vi "Initialize.vi"() -> (1 "Grid out":refnum<class "Grid.lvclass">, 2 "Synapses out":refnum<class "Synapses.lvclass">, 3 "Cerebellum out":refnum<class "Cerebellum.lvclass">, 4 "error out":errorcluster)   [LabVIEW 2016, in "Cerebellum.lvclass"]
doc: "Load/Create the flattened XML files for the Grid/Synapses/AER and plot it"
uses:
  Cerebellum.lvclass
  Cube/Grid.lvclass
  Controls/SM load Cere.ctl
  <vilib>/Utility/xml.llb/Read From XML File(string).vi
  Controls/Type of Neuron.ctl
  Synapses/Synapses.lvclass
  AER/AER.lvclass
  Neuron/Neuron.lvclass
panel:
  out "AER file path":path
  in  "Right":bool
  in  "Left":bool
  out "Syn ok?":bool
  in  "New AER":bool
  in  "Load AER":bool
  out "AER Loaded":string
  in  "3 - AER":i32(listbox)
  in  "Plot AER":bool
  in  "Plot Grid":bool
  in  "accept":bool
  out "Synapses Loaded":string
  out "Grid ok?":bool
  in  "New Synapses":bool
  in  "Load Synapses":bool
  in  "2 - Synapses":i32(listbox)
  out "Grid Loaded":string
  out "progress 2":dbl
  out "Preview":string
  in  "New Grid":bool
  in  "Cancel":bool
  in  "Load Grid":bool
  in  "1 - Grid":i32(listbox)
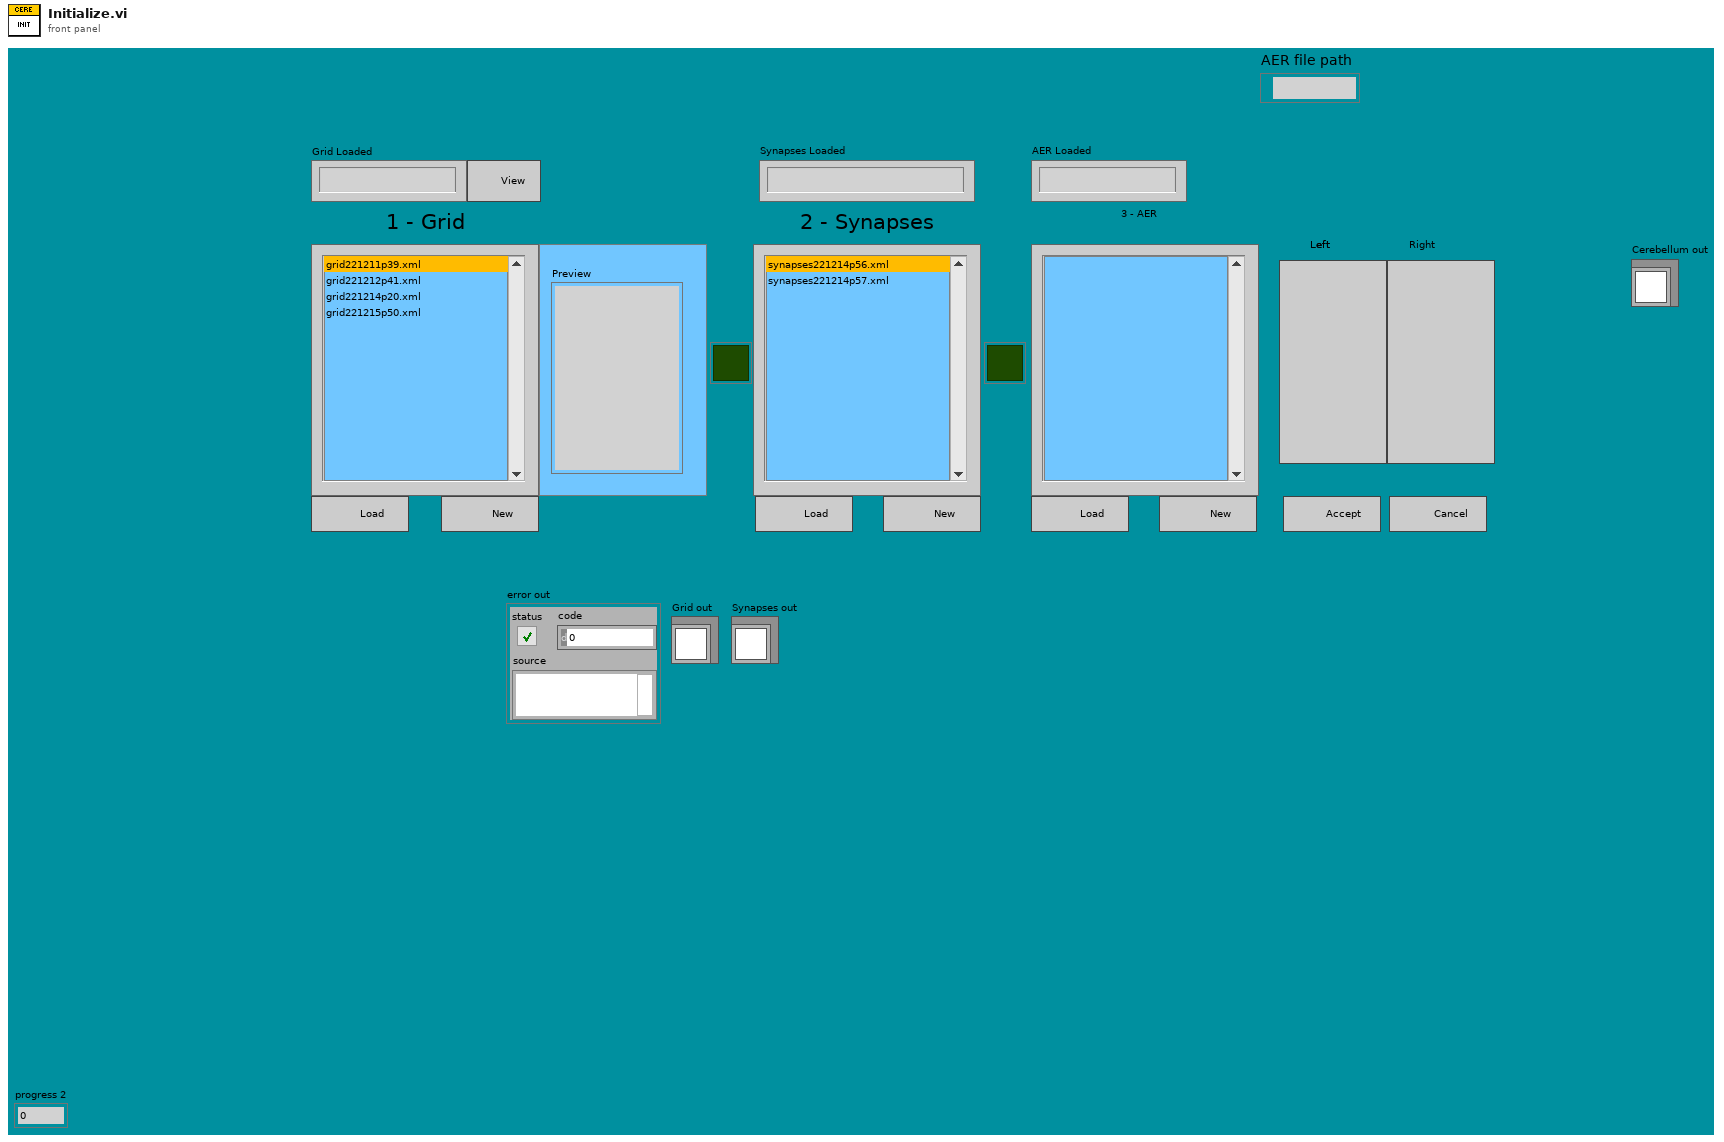
[diagram p1: front panel]
types:
  T1 = enum16{"open", "replace", "create", "open or create", "replace or create", "replace or create with confirmation"}
  T2 = typedef "SM load Cere.ctl" = enum16{"Create Grid", "Load Grid", "Create Synapses", "Load Synapses", "Cancel", "Update Lists", "accept", "Plot Grid", "Plot AER", "Load AER", "Create AER", "ToRightHem", "ToLeftHem"}
  T3 = typedef "Type of Neuron.ctl" = enum16{"MF", "BA", "GO", "GC", "PC", "LU", "Glia (Dummy)"}
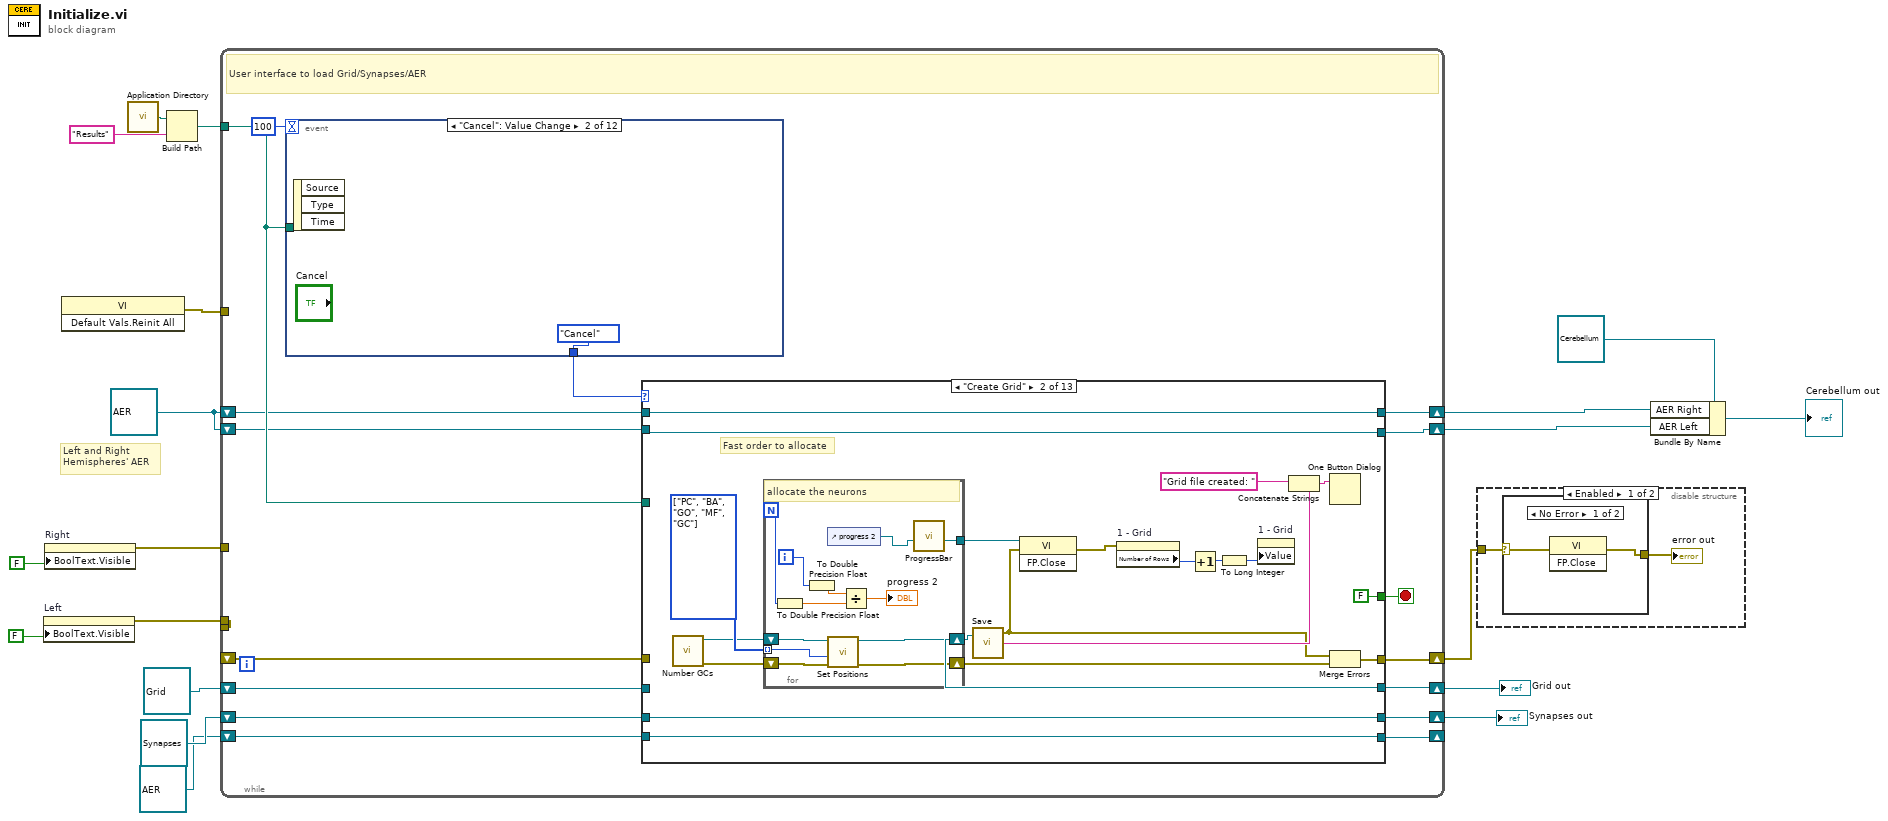
[diagram p0: block diagram]
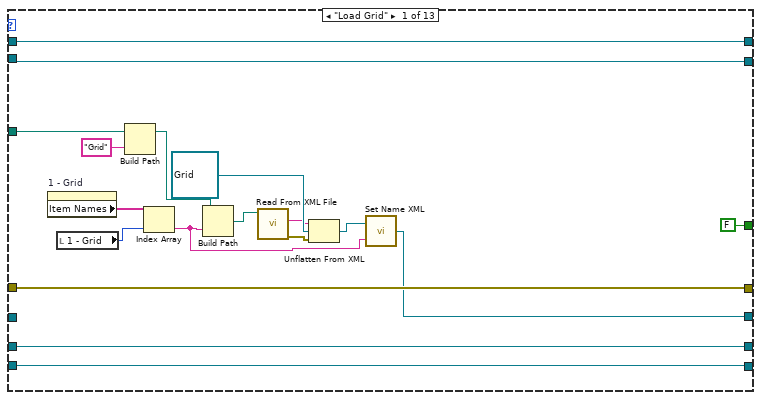
[diagram p4: hidden frame]
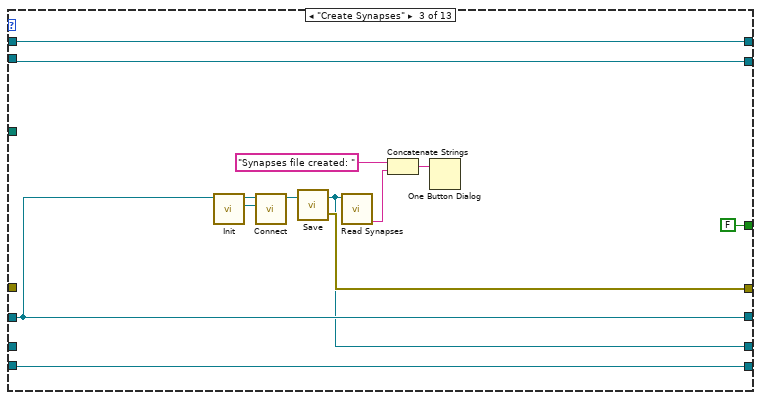
[diagram p5: hidden frame]
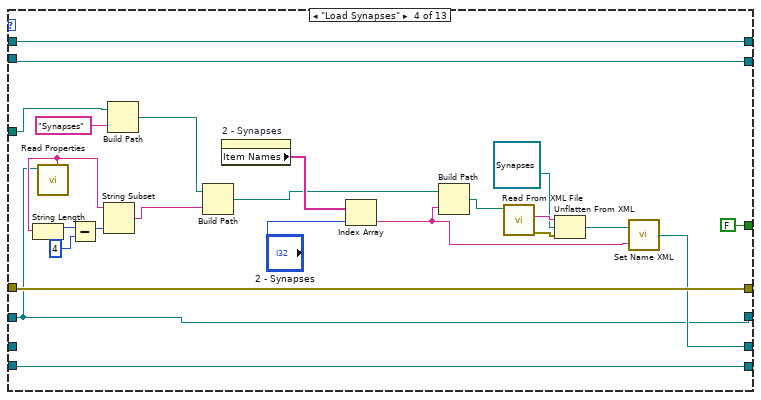
[diagram p6: hidden frame]
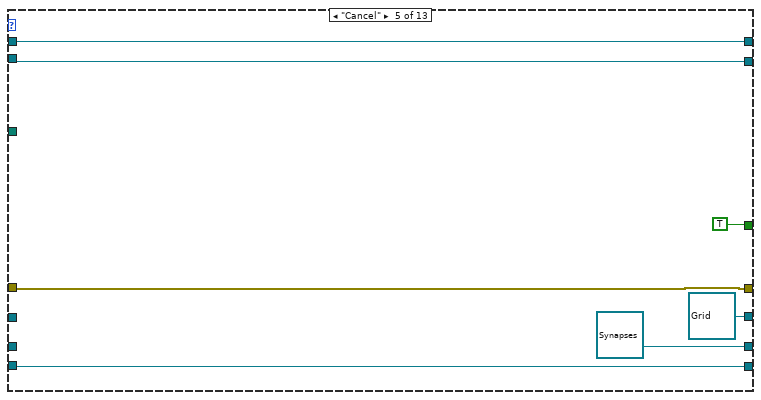
[diagram p7: hidden frame]
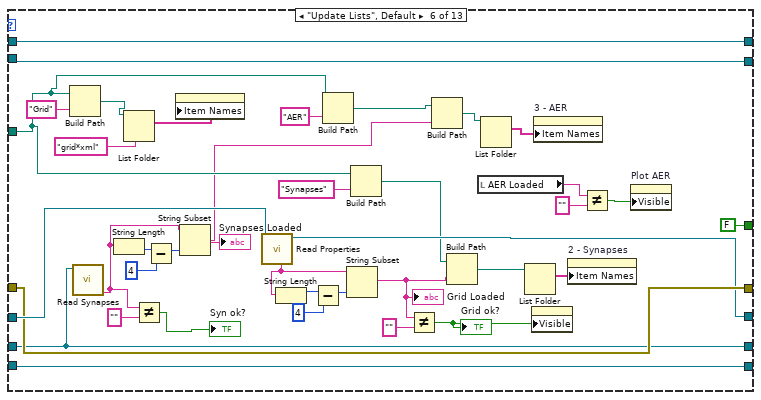
[diagram p8: hidden frame]
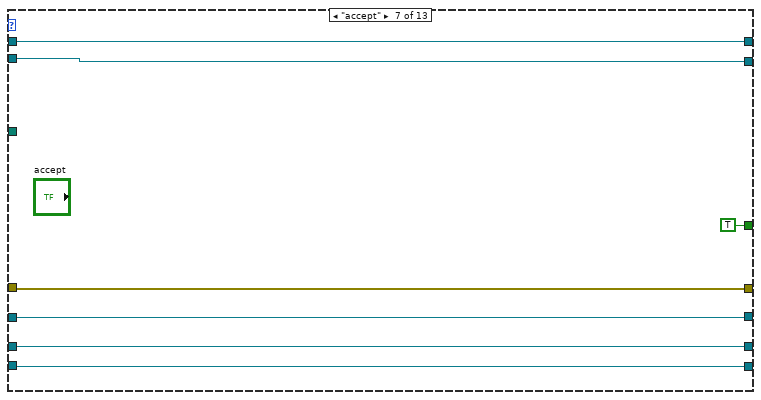
[diagram p9: hidden frame]
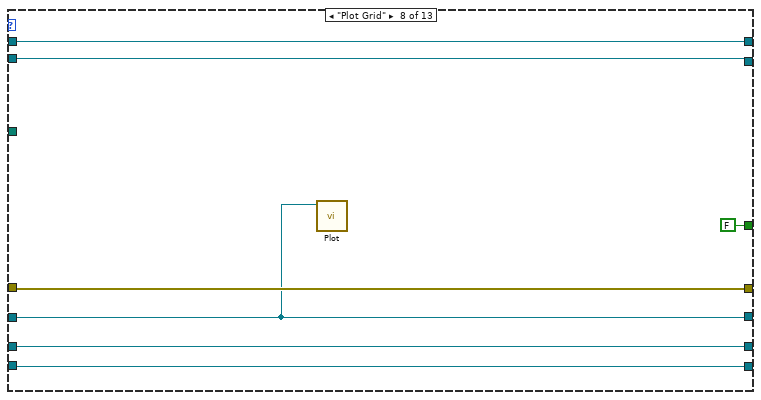
[diagram p10: hidden frame]
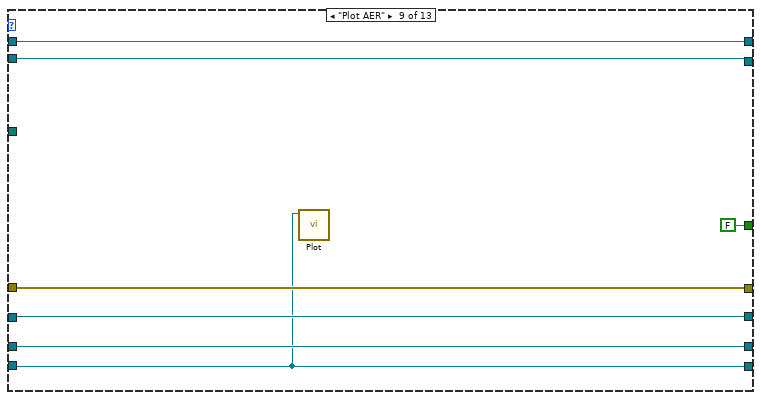
[diagram p11: hidden frame]
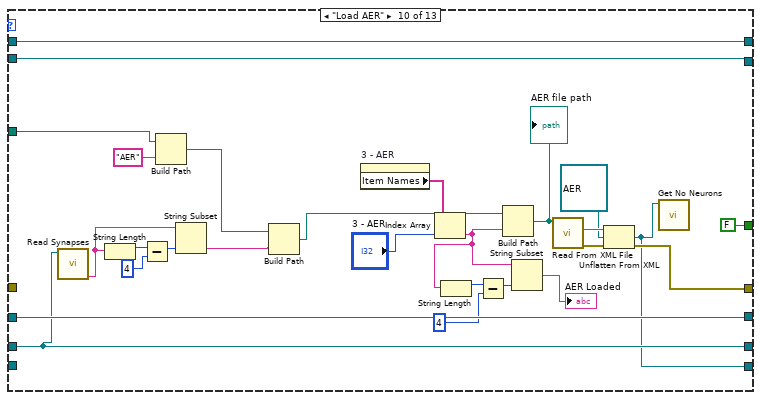
[diagram p12: hidden frame]
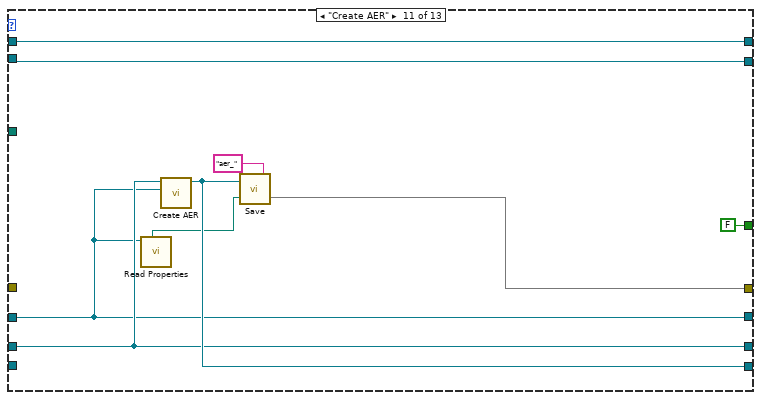
[diagram p13: hidden frame]
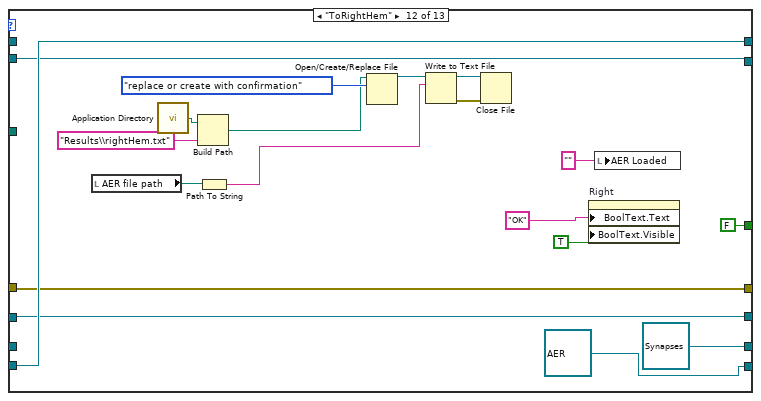
[diagram p14: hidden frame]
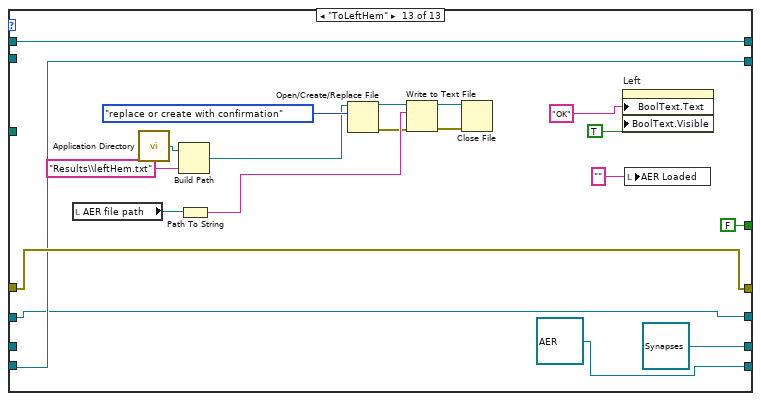
[diagram p15: hidden frame]
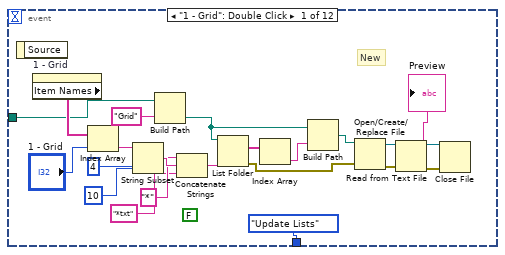
[diagram p16: hidden frame]
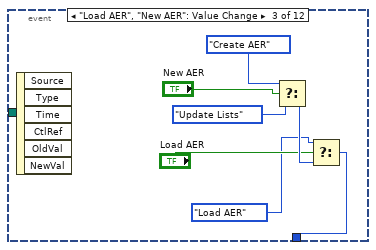
[diagram p17: hidden frame]
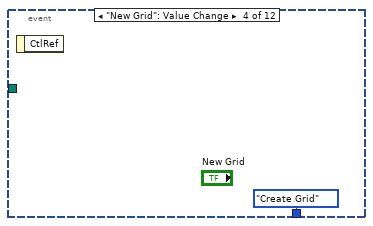
[diagram p18: hidden frame]
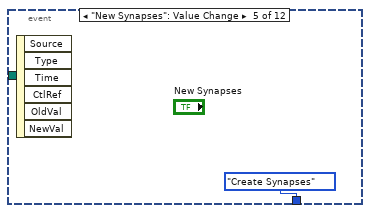
[diagram p19: hidden frame]
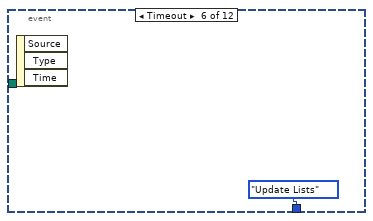
[diagram p20: hidden frame]
diagram:
  w9 = refnum<class "AER.lvclass"> refnum ("AER.lvclass")
  # "Left and Right\nHemispheres' AER"
  n1 = property on="Left" class="Bool (strict)"("BoolText.Visible"=FALSE ("Boolean Text.Visible")) -> (error out=w6:errorcluster)  [unwired: 2 in, 1 out]
  n2 = property on="Right" class="Bool (strict)"("BoolText.Visible"=FALSE ("Boolean Text.Visible")) -> (error out=w5:errorcluster)  [unwired: 2 in, 1 out]
  n3 = invoke class="VI" method="Default Vals.Reinit All"() -> (error out=w19:errorcluster)  [unwired: 3 in, 2 out]
  n4 = call <vilib>:"Application Directory.vi"() -> ("Application Directory"=w15:path)
  n5 = Build Path(base path=w15, name or relative path="Results") -> (appended path=w13:path)
  n6 = while {
    tunnel: w19 -> [_]
    shift-right: [w36] -> w18
    shift-left: refnum<class "Grid.lvclass"> refnum ("Cube out") -> [w33]
    shift-right: [w35] -> w16
    shift-left: _ -> [w34]
    tunnel: w13 -> [w32]
    shift-right: [w28] -> w11
    shift-left: refnum<class "Synapses.lvclass"> refnum ("Synapses out") -> [w27]
    shift-right: [w26] -> _
    shift-left: refnum<class "AER.lvclass"> refnum ("AER.lvclass") -> [w25]
    shift-right: [w22] -> w1
    shift-left: w9 -> [w21]
    shift-right: [w23] -> w2
    shift-left: w9 -> [w24]
    tunnel: [w20] -> _
    tunnel: w6 -> [w20]
    tunnel: w5 -> [_]
    stop <- w30 stop-if-true
    # "User interface to load Grid/Synapses/AER"
    n7 = event shown="[1] \"Cancel\": Value Change" {
      selector: _ -> [_ _ _ _ _ _ _ _ _ _ _ _]
      dyn-events: _ -> [_ _ _ _ _ _ _ _ _ _ _ _]
      timeout: 100 -> [_ _ _ _ _ _ _ _ _ _ _ _]
      tunnel: w32 -> [w268 _ _ _ _ _ _ _ _ _ _ _]
      tunnel: [SM_load_Cere."Update Lists" SM_load_Cere."Cancel" w288 SM_load_Cere."Create Grid" SM_load_Cere."Create Synapses" SM_load_Cere."Update Lists" SM_load_Cere."Load Synapses" SM_load_Cere."accept" w301 w307 SM_load_Cere."Load Grid" SM_load_Cere."Cancel"] -> w31
      event "1 - Grid": Double Click {
        (unwired) FALSE ("New")
        # "New"
        n8 = event-data() -> ()  [unwired: 1 in, 1 out]
        n9 = property on="1 - Grid" class="LstBox (strict)"() -> ("Item Names"=w286:string[])  [unwired: 2 in, 2 out]
        n10 = Index Array(array=w286, index="1 - Grid") -> (element=w269:string)
        n11 = String Subset(string=w269, offset (0)=4, length (rest)=10 ("length (rest)")) -> (substring=w283:string)
        n12 = Build Path(base path=w268, name or relative path="Grid") -> (appended path=w266:path)
        n13 = Concatenate Strings("*" ("string"), w283, "*txt" ("string")) -> (w282:string)
        n14 = List Folder(path=w266, pattern=w282) -> (filenames=w280:string[], error out=w276:errorcluster)  [unwired: 2 in, 2 out]
        n15 = Index Array(array=w280) -> (element=w279:string)  [unwired: 1 in]
        n16 = Build Path(base path=w266, name or relative path=w279) -> (appended path=w278:path)
        n17 = Open/Create/Replace File(file path (use dialog)=w278, error in=w276) -> (refnum out=w274:refnum<file>, error out=w275:errorcluster)  [unwired: 4 in, 1 out]
        n18 = Read from Text File(file (use dialog)=w274, error in=w275) -> (refnum out=w271:refnum<file>, text=→"Preview":string, error out=w272:errorcluster)  [unwired: 2 in, 1 out]
        n19 = Close File(refnum=w271, error in=w272) -> ()  [unwired: 2 out]
      }
      event "Cancel": Value Change {
        n20 = event-data() -> ()  [unwired: 1 in, 3 out]
      }
      event "Load AER", "New AER": Value Change {
        n21 = event-data() -> ()  [unwired: 1 in, 6 out]
        n22 = Select(t=SM_load_Cere."Create AER", s="New AER", f=SM_load_Cere."Update Lists") -> (s? t:f=w291:T2)
        n23 = Select(t=SM_load_Cere."Load AER", s="Load AER", f=w291) -> (s? t:f=w288:T2)
      }
      event "New Grid": Value Change {
        n24 = event-data() -> ()  [unwired: 1 in, 1 out]
      }
      event "New Synapses": Value Change {
        n25 = event-data() -> ()  [unwired: 1 in, 6 out]
      }
      event Timeout {
        n26 = event-data() -> ()  [unwired: 1 in, 3 out]
      }
      event "Load Synapses": Value Change {
        n27 = event-data() -> ()  [unwired: 1 in, 6 out]
      }
      event "accept": Value Change {
        n28 = event-data() -> ()  [unwired: 1 in, 6 out]
      }
      event "Plot AER", "Plot Grid": Value Change {
        n29 = event-data() -> ()  [unwired: 1 in, 6 out]
        n30 = Select(t=SM_load_Cere."Plot Grid", s="Plot Grid", f=SM_load_Cere."Update Lists") -> (s? t:f=w302:T2)
        n31 = Select(t=SM_load_Cere."Plot AER", s="Plot AER", f=w302) -> (s? t:f=w301:T2)
      }
      event "Left", "Right": Value Change {
        n32 = event-data() -> ()  [unwired: 1 in, 6 out]
        n33 = Select(t=SM_load_Cere."ToLeftHem", s="Left", f=SM_load_Cere."Update Lists") -> (s? t:f=w309:T2)
        n34 = Select(t=SM_load_Cere."ToRightHem", s="Right", f=w309) -> (s? t:f=w307:T2)
      }
      event "Load Grid": Value Change {
        n35 = event-data() -> ()  [unwired: 1 in, 1 out]
      }
      event Panel Close {
        # "The user closed the panel or selected \"Cancel.\""
        n36 = event-data() -> ()  [unwired: 1 in, 1 out]
      }
    }
    n37 = case shown="\"Create Grid\"" w31 {
      tunnel: [w43 w71 w91 w122 w128 w159 w174 w182 w189 w199 w223 w240 w261] -> w35
      tunnel: [w41 w67 w92 w108 refnum<class "Grid.lvclass"> refnum ("Cube out") w158 w173 w179 w188 w216 w219 w226 w245] -> w36
      tunnel: w33 -> [_ _ w92 w108 _ w160 w173 w179 w188 w216 w219 w226 w245]
      tunnel: w34 -> [w43 _ _ w122 w128 w159 w174 w182 w189 _ _ w240 w261]
      tunnel: w32 -> [w46 _ _ w109 _ w143 _ _ _ w204 _ _ _]
      tunnel: [FALSE FALSE FALSE FALSE TRUE FALSE TRUE FALSE FALSE FALSE FALSE FALSE FALSE] -> w30
      tunnel: [w44 w58 w90 w115 refnum<class "Synapses.lvclass"> refnum ("Synapses out") w156 w172 w181 w187 w209 w222 refnum<class "Synapses.lvclass"> refnum ("Synapses out") refnum<class "Synapses.lvclass"> refnum ("Synapses out")] -> w28
      tunnel: w27 -> [w44 w58 _ _ _ w156 w172 w181 w187 w209 w222 _ _]
      tunnel: [w42 w57 w89 w114 w126 w150 w171 w178 w185 w193 w225 refnum<class "AER.lvclass"> refnum ("AER.lvclass") refnum<class "AER.lvclass"> refnum ("AER.lvclass")] -> w26
      tunnel: w25 -> [w42 w57 w89 w114 w126 w150 w171 w178 w185 _ _ w244 w256]
      tunnel: w24 -> [w38 w56 w88 w101 w125 w132 w170 w177 w184 w192 w221 _ w264]
      tunnel: [w38 w56 w88 w101 w125 w132 w170 w177 w184 w192 w221 w244 w264] -> w23
      tunnel: [w37 w55 w87 w100 w124 w131 w169 w176 w183 w191 w220 w243 w256] -> w22
      tunnel: w21 -> [w37 w55 w87 w100 w124 w131 w169 w176 w183 w191 w220 w243 _]
      frame "Load Grid" {
        # "Load selected file"
        n38 = property on="1 - Grid" class="LstBox (strict)"() -> ("Item Names"=w53:string[])  [unwired: 2 in, 2 out]
        n39 = local read "1 - Grid"() -> (w49:i32)
        n40 = Build Path(base path=w46, name or relative path="Grid") -> (appended path=w40:path)
        n41 = Index Array(array=w53, index=w49) -> (element=w47:string)
        n42 = Build Path(base path=w40, name or relative path=w47) -> (appended path=w50:path)
        n43 = call-poly <vilib>:"Read From XML File.vi"("XML File Path"=w50) -> ("error out"=w51:errorcluster, "XML Elements"=w48:string)  [unwired: 8 in, 1 out]
        n44 = Unflatten From XML(xml string=w48, type=refnum<class "Grid.lvclass"> refnum ("Grid in"), error in (no error)=w51) -> (value=w54:refnum<class "Grid.lvclass">)  [unwired: 1 out]
        n45 = call-dynamic "Set Name XML.vi"("Name XML File"=w47, "Grid in"=w54) -> ("Grid out"=w41:refnum<class "Grid.lvclass">)
      }
      frame "Create Grid" {
        w74 = T3[] [enum."PC", enum."BA", enum."GO", enum."MF", enum."GC"] items=["MF", "BA", "GO", "GC", "PC", "LU", "Glia (Dummy)"]
        # "Fast order to allocate"
        # "Allocate neurons: New grid"
        n46 = call "Number GCs.vi"() -> ("error out"=w72:errorcluster, "Cube out"=w73:refnum<class "Grid.lvclass">)  [unwired: 5 in, 2 out]
        n47 = for {
          N -> [w81]
          shift-right: [w85] -> w67
          shift-left: w73 -> [w86]
          tunnel: w74 -> [w82] mode=indexing
          shift-right: [w83] -> w63
          shift-left: w72 -> [w84]
          tunnel: [w78] -> w66
          i -> [w77]
          # "allocate the neurons"
          n48 = To Double Precision Float(number=w81) -> (double precision float=w79:dbl)
          n49 = To Double Precision Float(number=w77) -> (double precision float=w80:dbl)
          n50 = control-ref of="progress 2"() -> (w75:refnum<vi>)
          n51 = call "Set Positions.vi"("error in"=w84, "Type of Neuron"=w82, "Grid in"=w86) -> ("error out"=w83:errorcluster, "Grid out"=w85:refnum<class "Grid.lvclass">)  [unwired: 7 in]
          n52 = Divide(x=w80, y=w79) -> (x/y=→"progress 2":dbl)
          n53 = call "ProgressBar.vi"("Progress"=w75) -> ("This VI"=w78:refnum<vi>)  [unwired: 10 in]
        }
        n54 = call "Save.vi"("Grid in"=w67) -> ("error out"=w65:errorcluster, "FileName"=w68:string)  [unwired: 1 in, 1 out]
        n55 = invoke class="VI" method="FP.Close"(reference=w66, error in=w65) -> (error out=w59:errorcluster)  [unwired: 1 in, 2 out]
        n56 = property on="1 - Grid" class="LstBox (strict)"(error in=w59) -> ("Number of Rows"=w64:u32)  [unwired: 1 in, 2 out]
        n57 = Increment(x=w64) -> (x+1=w62:u32)
        n58 = To Long Integer(number=w62) -> (32bit integer=w61:i32)
        n59 = property on="1 - Grid" class="LstBox (strict)"("Value"=w61) -> ()  [unwired: 2 in, 2 out]
        n60 = Concatenate Strings("Grid file created: " ("string"), w68) -> (w70:string)
        n61 = One Button Dialog(message=w70) -> ()  [unwired: 1 in, 1 out]
        n62 = Merge Errors(w65, w63) -> (w71:errorcluster)
      }
      frame "Create Synapses" {
        n63 = call "Init.vi"("Grid in"=w92) -> ("Grid out"=w98:refnum<class "Grid.lvclass">, "Synapses out"=w97:refnum<class "Synapses.lvclass">)  [unwired: 9 in]
        n64 = call "Connect.vi"("Grid in"=w98, "Synapses in"=w97) -> ("Synapses  out"=w94:refnum<class "Synapses.lvclass">)  [unwired: 8 in, 1 out]
        n65 = call "Save.vi"("Synapses in"=w94) -> ("error out"=w91:errorcluster, "Synapses out"=w90:refnum<class "Synapses.lvclass">)  [unwired: 1 in]
        n66 = call "Read Synapses.vi"("Synapses in"=w90) -> ("Name synapses File"=w93:string)  [unwired: 7 in, 3 out]
        n67 = Concatenate Strings("Synapses file created: " ("string"), w93) -> (w96:string)
        n68 = One Button Dialog(message=w96) -> ()  [unwired: 1 in, 1 out]
      }
      frame "Load Synapses" {
        n69 = call "Read Properties.vi"("Grid in"=w108) -> ("Name XML File"=w113:string)  [unwired: 3 in, 7 out]
        n70 = String Length(string=w113) -> (length=w112:i32)
        n71 = Subtract(x=w112, y=4 ("x")) -> (x-y=w111:i32)
        n72 = String Subset(string=w113, length (rest)=w111) -> (substring=w105:string)  [unwired: 1 in]
        n73 = Build Path(base path=w109, name or relative path="Synapses") -> (appended path=w106:path)
        n74 = Build Path(base path=w106, name or relative path=w105) -> (appended path=w104:path)
        n75 = property on="2 - Synapses" class="LstBox (strict)"() -> ("Item Names"=w116:string[])  [unwired: 2 in, 2 out]
        n76 = Index Array(array=w116, index="2 - Synapses") -> (element=w103:string)
        n77 = Build Path(base path=w104, name or relative path=w103) -> (appended path=w102:path)
        n78 = call-poly <vilib>:"Read From XML File.vi"("XML File Path"=w102) -> ("error out"=w120:errorcluster, "XML Elements"=w121:string)  [unwired: 8 in, 1 out]
        n79 = Unflatten From XML(xml string=w121, type=refnum<class "Synapses.lvclass"> refnum ("Synapses.lvclass"), error in (no error)=w120) -> (value=w118:refnum<class "Synapses.lvclass">)  [unwired: 1 out]
        n80 = call-dynamic "Set Name XML.vi"("Name XML File"=w103, "Synapses in"=w118) -> ("Synapses out"=w115:refnum<class "Synapses.lvclass">)
      }
      frame "Cancel" {
      }
      frame "Update Lists", Default {
        n81 = Build Path(base path=w143, name or relative path="Grid") -> (appended path=w149:path)
        n82 = call "Read Synapses.vi"("Synapses in"=w156) -> ("Name synapses File"=w151:string)  [unwired: 7 in, 3 out]
        n83 = String Length(string=w151) -> (length=w152:i32)
        n84 = List Folder(path=w149, pattern="grid*xml") -> (filenames=w167:string[])  [unwired: 2 in, 3 out]
        n85 = Not Equal?(x=w151, y="") -> (x != y?=→"Syn ok?":bool)
        n86 = Subtract(x=w152, y=4 ("x")) -> (x-y=w153:i32)
        n87 = property on="1 - Grid" class="LstBox (strict)"("Item Names"=w167) -> ()  [unwired: 2 in, 2 out]
        n88 = String Subset(string=w151, length (rest)=w153) -> (substring=w138:string)  [unwired: 1 in]
        "Synapses Loaded" <- w138
        n89 = call "Read Properties.vi"("Grid in"=w160) -> ("Grid out"=w158:refnum<class "Grid.lvclass">, "Name XML File"=w164:string)  [unwired: 3 in, 6 out]
        n90 = String Length(string=w164) -> (length=w163:i32)
        n91 = Subtract(x=w163, y=4 ("x")) -> (x-y=w162:i32)
        n92 = Build Path(base path=w143, name or relative path="AER") -> (appended path=w139:path)
        n93 = String Subset(string=w164, length (rest)=w162) -> (substring=w142:string)  [unwired: 1 in]
        "Grid Loaded" <- w142
        n94 = Build Path(base path=w143, name or relative path="Synapses") -> (appended path=w141:path)
        n95 = Not Equal?(x=w142, y="") -> (x != y?=w137:bool)
        "Grid ok?" <- w137
        n96 = Build Path(base path=w139, name or relative path=w138) -> (appended path=w145:path)
        n97 = Build Path(base path=w141, name or relative path=w142) -> (appended path=w140:path)
        n98 = local read "AER Loaded"() -> (w135:string)
        n99 = List Folder(path=w145) -> (filenames=w144:string[])  [unwired: 3 in, 3 out]
        n100 = List Folder(path=w140) -> (filenames=w165:string[])  [unwired: 3 in, 3 out]
        n101 = property on="Plot Grid" class="Bool"("Visible"=w137) -> ()  [unwired: 2 in, 2 out]
        n102 = property on="3 - AER" class="LstBox (strict)"("Item Names"=w144) -> ()  [unwired: 2 in, 2 out]
        n103 = property on="2 - Synapses" class="LstBox (strict)"("Item Names"=w165) -> ()  [unwired: 2 in, 2 out]
        n104 = Not Equal?(x=w135, y="") -> (x != y?=w134:bool)
        n105 = property on="Plot AER" class="Bool"("Visible"=w134) -> ()  [unwired: 2 in, 2 out]
      }
      frame "accept" {
      }
      frame "Plot Grid" {
        n106 = call "Plot.vi"("Grid in"=w179) -> ()  [unwired: 11 in]
      }
      frame "Plot AER" {
        n107 = call "Plot.vi"("AER in"=w185) -> ()  [unwired: 11 in]
      }
      frame "Load AER" {
        n108 = call "Read Synapses.vi"("Synapses in"=w209) -> ("Name synapses File"=w205:string)  [unwired: 7 in, 3 out]
        n109 = String Length(string=w205) -> (length=w208:i32)
        n110 = Subtract(x=w208, y=4 ("x")) -> (x-y=w207:i32)
        n111 = Build Path(base path=w204, name or relative path="AER") -> (appended path=w201:path)
        n112 = String Subset(string=w205, length (rest)=w207) -> (substring=w202:string)  [unwired: 1 in]
        n113 = Build Path(base path=w201, name or relative path=w202) -> (appended path=w200:path)
        n114 = property on="3 - AER" class="LstBox (strict)"() -> ("Item Names"=w210:string[])  [unwired: 2 in, 2 out]
        n115 = Index Array(array=w210, index="3 - AER") -> (element=w194:string)
        n116 = String Length(string=w194) -> (length=w196:i32)
        n117 = Subtract(x=w196, y=4 ("x")) -> (x-y=w197:i32)
        n118 = Build Path(base path=w200, name or relative path=w194) -> (appended path=w190:path)
        "AER file path" <- w190
        n119 = String Subset(string=w194, length (rest)=w197) -> (substring=→"AER Loaded":string)  [unwired: 1 in]
        n120 = call-poly <vilib>:"Read From XML File.vi"("XML File Path"=w190) -> ("error out"=w213:errorcluster, "XML Elements"=w214:string)  [unwired: 8 in, 1 out]
        n121 = Unflatten From XML(xml string=w214, type=refnum<class "AER.lvclass"> refnum ("AER.lvclass"), error in (no error)=w213) -> (value=w193:refnum<class "AER.lvclass">, error out=w199:errorcluster)
        n122 = call "Get No Neurons.vi"("AER in"=w193) -> ()  [unwired: 9 in, 2 out]
      }
      frame "Create AER" {
        n123 = call "Read Properties.vi"("Grid in"=w219) -> ("Path"=w218:path)  [unwired: 3 in, 7 out]
        n124 = call "Create AER.vi"("Grid.lvclass"=w219, "Synapses in"=w222) -> ("AER.lvclass"=w225:refnum<class "AER.lvclass">)  [unwired: 6 in, 3 out]
        n125 = call "Save.vi"("AER file name"="aer_", "Inpath"=w218, "AER in"=w225) -> (0:w223)
      }
      frame "ToRightHem" {
        n126 = local read "AER file path"() -> (w230:path)
        n127 = call <vilib>:"Application Directory.vi"() -> ("Application Directory"=w233:path)
        n128 = Build Path(base path=w233, name or relative path="Results\\rightHem.txt") -> (appended path=w231:path)
        n129 = Path To String(path=w230) -> (string=w229:string)
        n130 = Open/Create/Replace File(file path (use dialog)=w231, operation (0:open)=T1."replace or create with confirmation") -> (refnum out=w234:refnum<file>)  [unwired: 4 in, 2 out]
        n131 = Write to Text File(file (use dialog)=w234, text=w229) -> (refnum out=w227:refnum<file>, error out=w228:errorcluster)  [unwired: 2 in, 1 out]
        n132 = Close File(refnum=w227, error in=w228) -> ()  [unwired: 2 out]
        n133 = property on="Right" class="Bool (strict)"("BoolText.Text"="OK" ("Boolean Text.Text"), "BoolText.Visible"=TRUE ("Boolean Text.Visible")) -> ()  [unwired: 2 in, 2 out]
        n134 = local write "AER Loaded"("" ("AER Loaded")) -> ()
      }
      frame "ToLeftHem" {
        n135 = local read "AER file path"() -> (w250:path)
        n136 = call <vilib>:"Application Directory.vi"() -> ("Application Directory"=w253:path)
        n137 = Build Path(base path=w253, name or relative path="Results\\leftHem.txt") -> (appended path=w251:path)
        n138 = Path To String(path=w250) -> (string=w249:string)
        n139 = Open/Create/Replace File(file path (use dialog)=w251, operation (0:open)=T1."replace or create with confirmation") -> (refnum out=w254:refnum<file>, error out=w246:errorcluster)  [unwired: 4 in, 1 out]
        n140 = Write to Text File(file (use dialog)=w254, text=w249, error in=w246) -> (refnum out=w247:refnum<file>, error out=w248:errorcluster)  [unwired: 1 in, 1 out]
        n141 = Close File(refnum=w247, error in=w248) -> ()  [unwired: 2 out]
        n142 = property on="Left" class="Bool (strict)"("BoolText.Text"="OK" ("Boolean Text.Text"), "BoolText.Visible"=TRUE ("Boolean Text.Visible")) -> ()  [unwired: 2 in, 2 out]
        n143 = local write "AER Loaded"("" ("AER Loaded")) -> ()
      }
    }
  }
  "Grid out" <- w18
  "Synapses out" <- w11
  n144 = disable-structure shown="Enabled" {
    disable-tunnel: w16 -> [w316 _]
    frame Enabled {
      n145 = case shown="No Error" w316 {
        selector: w316 -> [w319 w320]
        tunnel: [w318 w320] -> w317
        frame No Error {
          n146 = invoke on="Invoke Node" class="VI" method="FP.Close"(error in=w319) -> (error out=w318:errorcluster)  [unwired: 2 in, 2 out]
        }
        frame Error {
        }
      }
      "error out" <- w317
    }
    frame Disabled {
    }
  }
  n147 = Bundle By Name(cluster=refnum<class "Cerebellum.lvclass"> refnum ("Cerebellum in"), "AER Right"=w2, "AER Left"=w1) -> (→"Cerebellum out":refnum<class "Cerebellum.lvclass">)
